vi "Hardware-Skipfire-Host.vi"() -> ()   [LabVIEW 2016]
uses:
  <vilib>/Powertrain Controls/Device Drivers/DCM/Skip Fire/RT/Skip Fire Setup.ctl
  <vilib>/Powertrain Controls/Device Drivers/DCM/Skip Fire/RT/DCM - RT - Skip Fire.lvlib
panel:
  in  "_Hidden":enum32{"Page 1"}(tab)
  in  "_Refresh":bool
  in  "Setup":T1[](array[typedef])
  in  "AdaptMode":u32
  in  "ChannelNames":string
  in  "_Skipfire Channels":i32(listbox) caption="Summary"
  in  "_Name":string caption="Name"
  in  "_AdaptMode":bool caption="Adapt Mode"
  in  "_Skipfire Settings":T1 caption="Settings"
  # "Skipfire Settings"
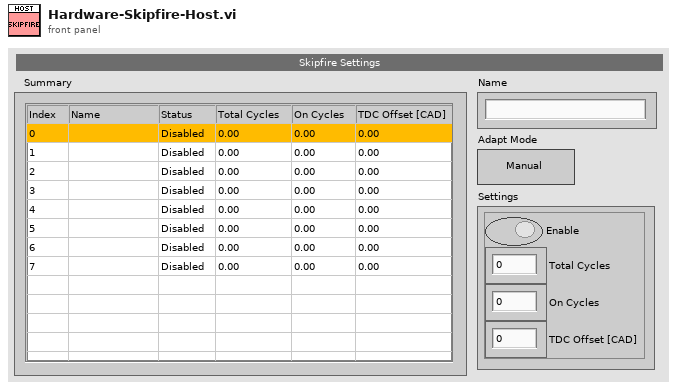
[diagram p1: front panel]
types:
  T1 = typedef "DCM - RT - Skip Fire.lvlib/Skip Fire Setup.ctl" = cluster{"Enable":bool, "Total Cycles":u8, "On Cycles":u8, "TDC Offset [CAD]":sgl}
  T2 = enum8{"Enabled", "Disabled", "Disabled and Grayed Out"}
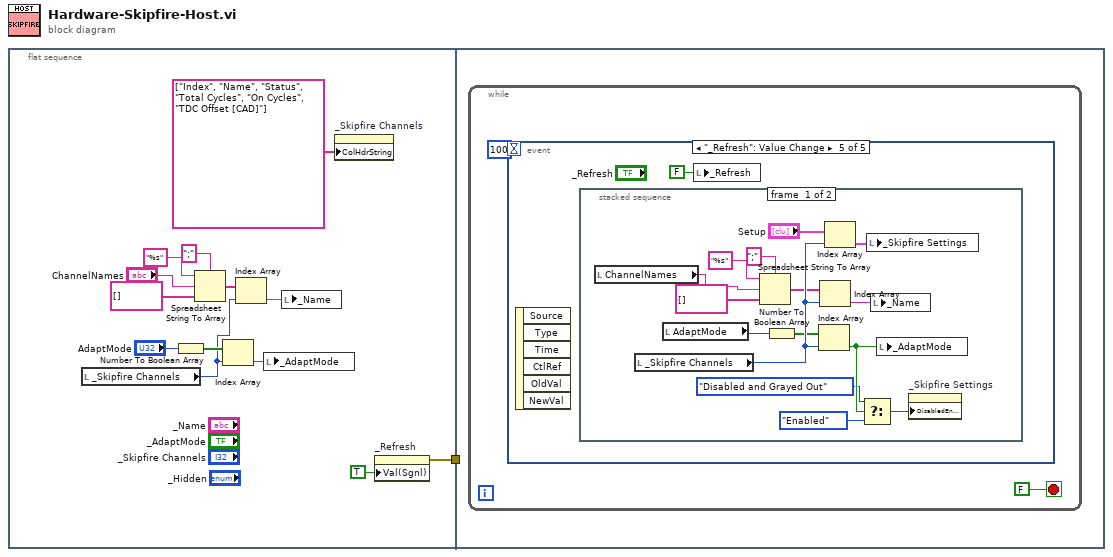
[diagram p0: block diagram]
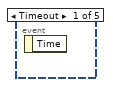
[diagram p2: hidden frame]
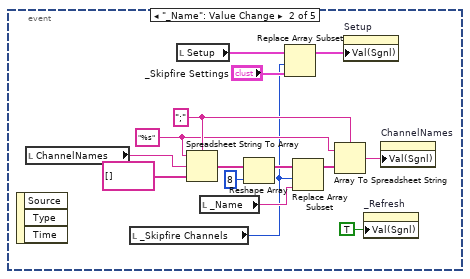
[diagram p3: hidden frame]
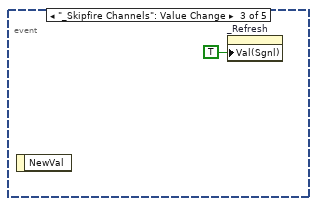
[diagram p4: hidden frame]
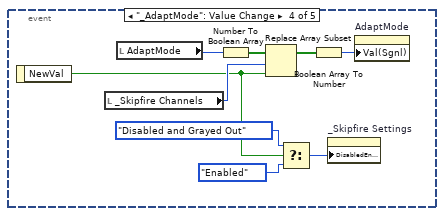
[diagram p5: hidden frame]
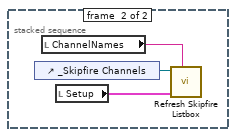
[diagram p6: hidden frame]
diagram:
  n1 = flat-sequence {
    tunnel: [w2] -> w1
    tunnel: w1 -> [_]
    frame #0 {
      n2 = local read "_Skipfire Channels"() -> (w5:i32)
      n3 = Number To Boolean Array(number="AdaptMode") -> (Boolean array=w11:bool[])
      n4 = Spreadsheet String To Array(delimiter (Tab)=";", format string="%s" ("spreadsheet string"), spreadsheet string="ChannelNames", array type (2D Dbl)=string[] [] ("ChannelNames")) -> (array=w7:string[])
      n5 = Index Array(array=w11, index=w5) -> (element=w10:bool)
      n6 = Index Array(array=w7, index=w5) -> (element=w6:string)
      n7 = local write "_AdaptMode"(w10) -> ()
      n8 = local write "_Name"(w6) -> ()
      n9 = property on="_Skipfire Channels" class="MCListbox (strict)"("ColHdrString"=string[] ["Index", "Name", "Status", "Total Cycles", "On Cycles", "TDC Offset [CAD]"] ("Column Header Strings[] 2")) -> ()  [unwired: 2 in, 2 out]
      n10 = property on="_Refresh" class="Bool (strict)"("Val(Sgnl)"=TRUE ("Value (Signaling)")) -> (error out=w2:errorcluster)  [unwired: 2 in, 1 out]
    }
    frame #1 {
      n11 = while {
        stop <- FALSE stop-if-true
        n12 = event shown="[4] \"_Refresh\": Value Change" {
          selector: _ -> [_ _ _ _ _]
          dyn-events: _ -> [_ _ _ _ _]
          timeout: 100 -> [_ _ _ _ _]
          event Timeout {
            n13 = event-data() -> ()  [unwired: 1 in, 1 out]
          }
          event "_Name": Value Change {
            w20 = "%s" ("spreadsheet string")
            w23 = ";" ("delimiter (Tab)")
            n14 = event-data() -> ()  [unwired: 1 in, 3 out]
            n15 = local read "ChannelNames"() -> (w21:string)
            n16 = local read "_Skipfire Channels"() -> (w17:i32)
            n17 = local read "Setup"() -> (w30:T1[])
            n18 = Spreadsheet String To Array(delimiter (Tab)=w23, format string=w20, spreadsheet string=w21, array type (2D Dbl)=string[] [] ("ChannelNames")) -> (array=w25:string[])
            n19 = local read "_Name"() -> (w27:string)
            n20 = Reshape Array(w25, 8 ("dimension size")) -> (w19:string[])
            n21 = Replace Array Subset(array=w30, new element="_Skipfire Settings", index=w17) -> (w29:T1[])
            n22 = Replace Array Subset(array=w19, new element=w27, index=w17) -> (w24:string[])
            n23 = Array To Spreadsheet String(delimiter (Tab)=w23, array=w24, 3:w20) -> (spreadsheet string=w22:string)
            n24 = property on="Setup" class="Arr (strict)"("Val(Sgnl)"=w29) -> ()  [unwired: 2 in, 2 out]
            n25 = property on="_Refresh" class="Bool (strict)"("Val(Sgnl)"=TRUE ("Value (Signaling)")) -> ()  [unwired: 2 in, 2 out]
            n26 = property on="ChannelNames" class="Str"("Val(Sgnl)"=w22) -> ()  [unwired: 2 in, 2 out]
          }
          event "_Skipfire Channels": Value Change {
            n27 = event-data() -> ()  [unwired: 1 in, 1 out]
            n28 = property on="_Refresh" class="Bool (strict)"("Val(Sgnl)"=TRUE ("Value (Signaling)")) -> ()  [unwired: 2 in, 2 out]
          }
          event "_AdaptMode": Value Change {
            n29 = event-data() -> ("NewVal"=w34:bool)  [unwired: 1 in]
            n30 = local read "_Skipfire Channels"() -> (w37:i32)
            n31 = local read "AdaptMode"() -> (w40:u32)
            n32 = Number To Boolean Array(number=w40) -> (Boolean array=w41:bool[])
            n33 = Replace Array Subset(array=w41, new element=w34, index=w37) -> (w39:bool[])
            n34 = Select(t=T2."Disabled and Grayed Out" ("Disabled"), s=w34, f=T2."Enabled" ("Disabled")) -> (s? t:f=w33:T2)
            n35 = Boolean Array To Number(Boolean array=w39) -> (number=w38:u32)
            n36 = property on="_Skipfire Settings" class="Clust (strict)"("DisabledEnum"=w33) -> ()  [unwired: 2 in, 2 out]
            n37 = property on="AdaptMode" class="DigNum (strict)"("Val(Sgnl)"=w38) -> ()  [unwired: 2 in, 2 out]
          }
          event "_Refresh": Value Change {
            n38 = event-data() -> ()  [unwired: 1 in, 6 out]
            n39 = stacked-sequence {
              frame #0 {
                n40 = local read "ChannelNames"() -> (w47:string)
                n41 = local read "_Skipfire Channels"() -> (w53:i32)
                n42 = local read "AdaptMode"() -> (w45:u32)
                n43 = Spreadsheet String To Array(delimiter (Tab)=";", format string="%s" ("spreadsheet string"), spreadsheet string=w47, array type (2D Dbl)=string[] [] ("ChannelNames")) -> (array=w46:string[])
                n44 = Number To Boolean Array(number=w45) -> (Boolean array=w44:bool[])
                n45 = Index Array(array=w44, index=w53) -> (element=w57:bool)
                n46 = Index Array(array=w46, index=w53) -> (element=w43:string)
                n47 = Index Array(array="Setup", index=w53) -> (element=w52:T1)
                n48 = Select(t=T2."Disabled and Grayed Out" ("Disabled"), s=w57, f=T2."Enabled" ("Disabled")) -> (s? t:f=w54:T2)
                n49 = local write "_Skipfire Settings"(w52) -> ()
                n50 = local write "_Name"(w43) -> ()
                n51 = local write "_AdaptMode"(w57) -> ()
                n52 = property on="_Skipfire Settings" class="Clust (strict)"("DisabledEnum"=w54) -> ()  [unwired: 2 in, 2 out]
              }
              frame #1 {
                n53 = control-ref of="_Skipfire Channels"() -> (w60:refnum<vi>)
                n54 = local read "ChannelNames"() -> (w58:string)
                n55 = local read "Setup"() -> (w59:T1[])
                n56 = call "Refresh Skipfire Listbox.vi"("ChannelNames"=w58, "IRQ Settings Array"=w59, "IRQ Listbox Refnum"=w60) -> ()  [unwired: 9 in]
              }
            }
            n57 = local write "_Refresh"(FALSE ("_Refresh")) -> ()
          }
        }
      }
    }
  }
